vi "TCP Client_34_enablep.vi"(0 "CMD":i32(ring) items=["OCP_IF_CMD_TRACE_READ", "OCP_IF_CMD_TRACE_RESET", "OCP_IF_CMD_TRACE_GET_SIZE", "OCP_IF_CMD_TRACE_SET_SIZE", "OCP_IF_CMD_TRACE_GET_NUMBER_SIGNALS", "OCP_IF_CMD_TRACE_GET_SIGNALS_NAMES", "OCP_IF_CMD_TRACE_GET_NUMBER_TRACES", "OCP_IF_CMD_TRACE_GET_TRACES_NAMES", "OCP_IF_CMD_TRACE_GET_ADDRESS", "OCP_IF_CMD_CS_STATUS", "OCP_IF_CMD_CS_ENABLE", "OCP_IF_CMD_CS_DISABLE", "OCP_IF_CMD_CS_CONTROLLER_IF", "OCP_IF_CMD_CS_HARDWARE_IF", "OCP_IF_CMD_CS_GET_NUMBER_CONTROLLERS", "OCP_IF_CMD_CS_GET_CONTROLLERS_NAMES", "OCP_IF_CMD_PLATFORM_ID", "OCP_IF_CMD_PLATFORM_IF", "OCP_IF_CMD_OPIL_UPDATE_MEASUREMENTS", "OCP_IF_CMD_OPIL_UPDATE_SIM_DATA", "OCP_IF_CMD_OPIL_RUN_CONTROL", "OCP_IF_CMD_OPIL_INITIALIZE_CONTROL", "OCP_IF_CMD_OPIL_GET_CONTROL", "OCP_IF_CMD_OPIL_GET_CONTROLLER_DATA", "OCP_IF_CMD_END"], 1 "CS_IF_Params":T1 {"CS_Duty" min=0 max=1}, 2 "Input Cluster":T4, 3 "error in (no error)":errorcluster, 8 "Comunication Cluster":T2) -> (6 "Output cluster":T3, 7 "R_message 1":string, 10 "error out":errorcluster)   [LabVIEW 2021]
uses:
  <vilib>/ErrorRing/Error Ring.xnode
  <vilib>/Utility/error.llb/Error Cluster From Error Code.vi
panel:
  out "R_Data string length":cluster{i32}
  out "W_Data string length: \nbytes written 2":i32
  out "W_Data string_flat":string
  # "0-> OCP_IF_CMD_TRACE_READ = 0, //LV: SIZE - CMD - ID || RESPONSE: SIZE - DATA\n1->\tOCP_IF_CMD_TRACE_RESET, //SIZE - CMD - ID || RESPONSE: SIZE\n2-> OCP_IF_CMD_TRACE_GET_SIZE, //SIZE - CMD - ID || RESPONSE: SIZE - TRACE_SIZE (4 bztes)\n3->\tOCP_IF_CMD_TRACE_SET_SIZE, //SIZE - CMD - ID - TRACE_SIZE ( 4 bytes) || RESPONSE: SIZE\n4->\tOCP_IF_CMD_TRACE_GET_NUMBER_SIGNALS, //SIZE - CMD - ID || RESPONSE: SIZE - NB_SIGNALS (4 bytes)\n5->\tOCP_IF_CMD_TRACE_GET_SIGNALS_NAMES, //SIZE - CMD - ID || RESPONSE: SIZE - string\n6->\tOCP_IF_CMD_TRACE_GET_NUMBER_TRACES, //SIZE - CMD  || RESPONSE: SIZE - NB_TRACES (4 bytes)\n7->\tOCP_IF_CMD_TRACE_GET_TRACES_NAMES, //SIZE - CMD || RESPONSE: SIZE - NB_TRACES (N bytes)\n8-> OCP_IF_CMD_TRACE_GET_ADDRESS, //SIZE - CMD - ID || RESPONSE: SIZE - TRACE ADDRESS (4 bytes)\n9-> OCP_IF_CMD_CS_STATUS, //SIZE - CMD - ID || RESPONSE: SIZE - CS STATUS (4 bytes)\n10-> OCP_IF_CMD_CS_ENABLE, //SIZE - CMD - ID || RESPONSE: SIZE\n11-> OCP_IF_CMD_CS_DISABLE, //SIZE - CMD - ID || RESPONSE: SIZE\n12-> OCP_IF_CMD_CS_CONTROLLER_IF, //SIZE - CMD - ID - DATA (N) || RESPONSE: SIZE - DATA (M)\n13-> OCP_IF_CMD_CS_HARDWARE_IF, //SIZE - CMD - ID - DATA (N) || RESPONSE: SIZE - DATA (M)\n14-> OCP_IF_CMD_CS_GET_NUMBER_CONTROLLERS, //SIZE - CMD || RESPONSE: SIZE - NB CSs\n15-> OCP_IF_CMD_CS_GET_CONTROLLERS_NAMES, //SIZE - CMD || RESPONSE: SIZE - string NAMES CSs"
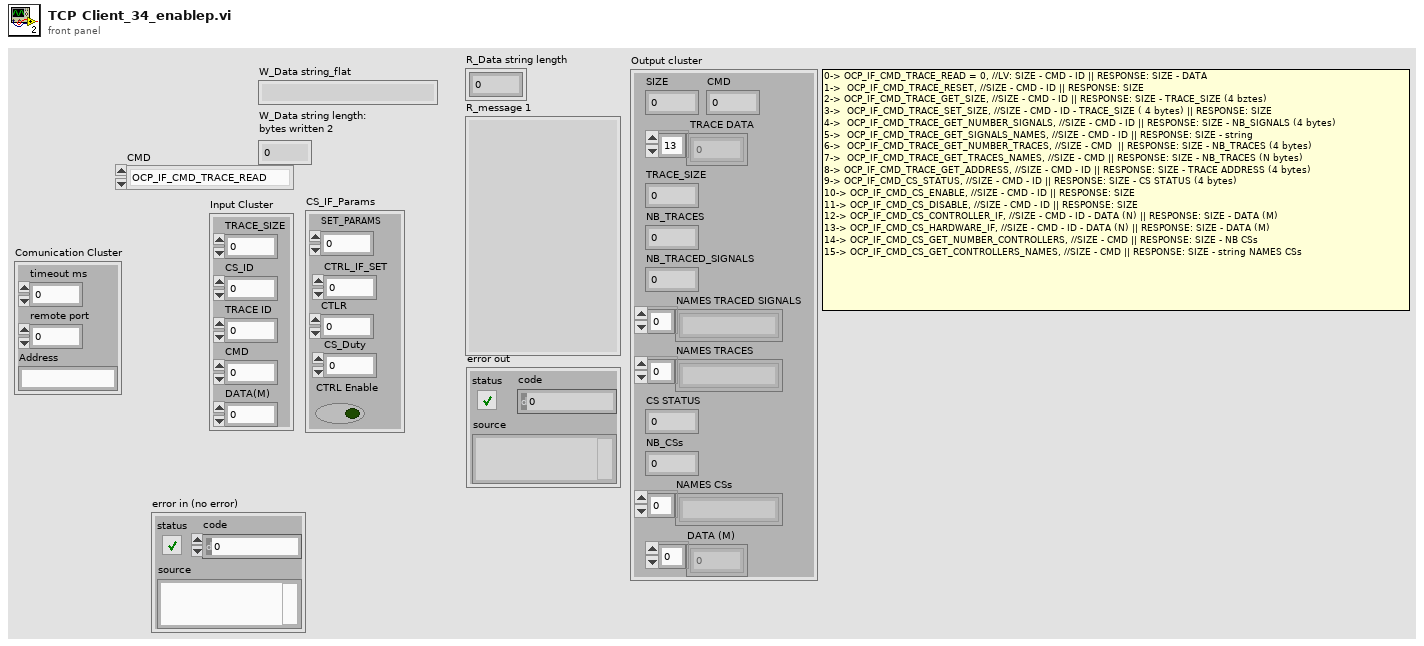
[diagram p1: front panel]
types:
  T1 = cluster{"SET_PARAMS":i32, "CTLR":i32, "CS_Duty":sgl, "CTRL_IF_SET":i32, "CTRL Enable":bool}
  T2 = cluster{"timeout ms":i32, "remote port":u16, "Address":string}
  T3 = cluster{"SIZE":i32, " TRACE DATA":sgl[], "TRACE_SIZE":i32, "NB_TRACES":i32, "NB_TRACED_SIGNALS":i32, "NAMES TRACED SIGNALS":string[], "NAMES TRACES":string[], "CS STATUS":i32, "NB_CSs":i32, "NAMES CSs":string[], "DATA (M)":sgl[], "CMD":i32}
  T4 = cluster{"TRACE_SIZE":i32, "CS_ID":i32, "TRACE ID":i32, "CMD":i32, "DATA(M)":i32}
  T5 = enum16{"big-endian, network order", "native, host order", "little-endian"}
  T6 = enum16{"Standard", "Buffered", "CRLF", "Immediate"}
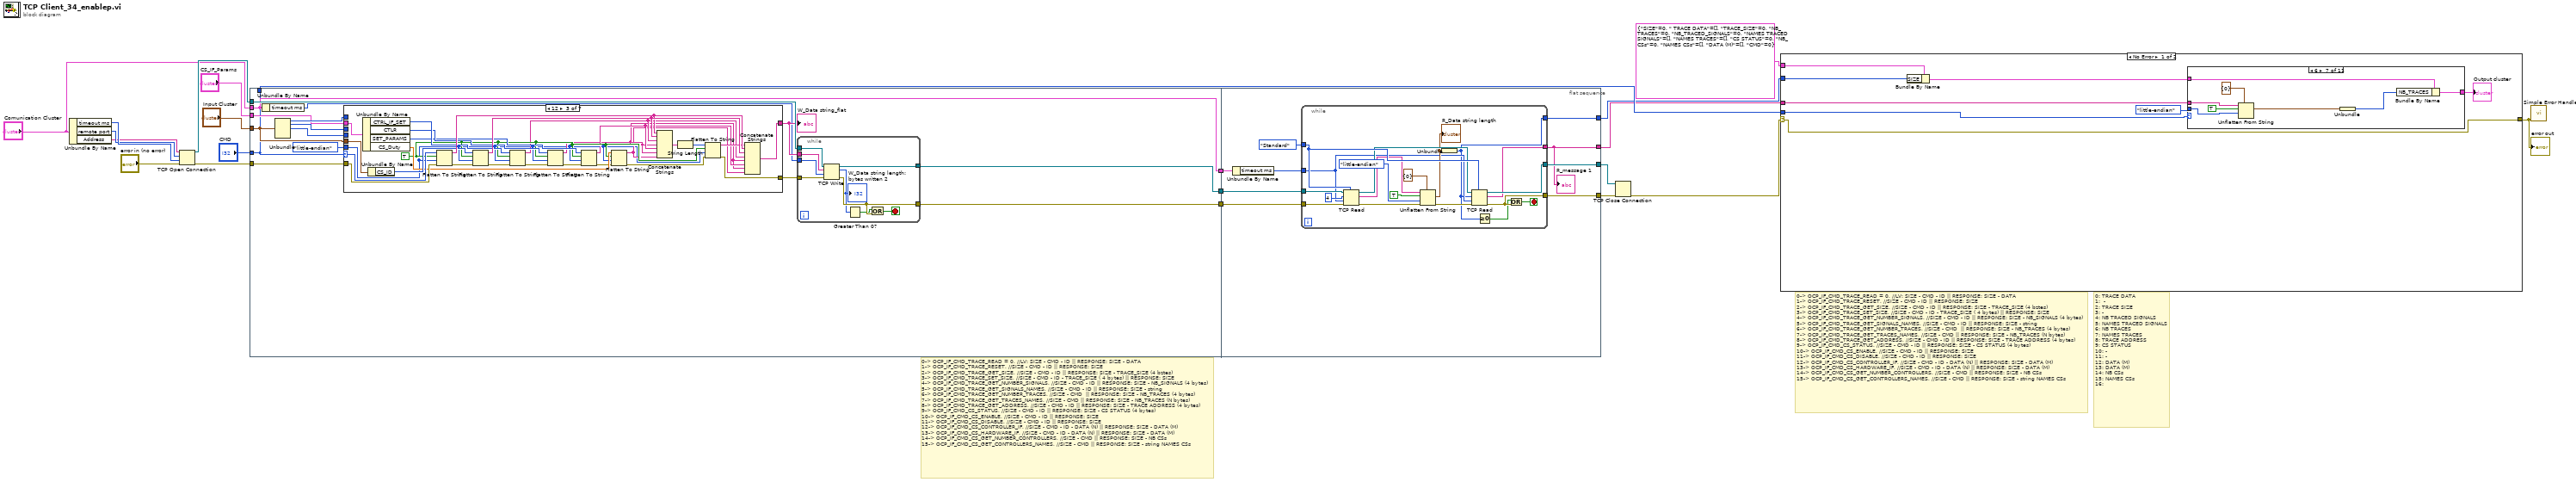
[diagram p0: block diagram]
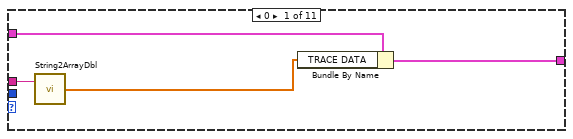
[diagram p2: hidden frame]
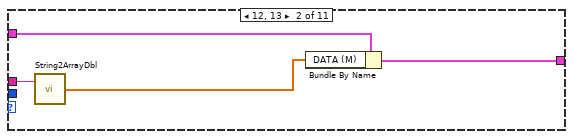
[diagram p3: hidden frame]
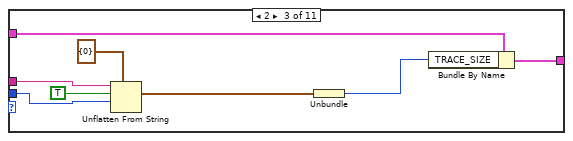
[diagram p4: hidden frame]
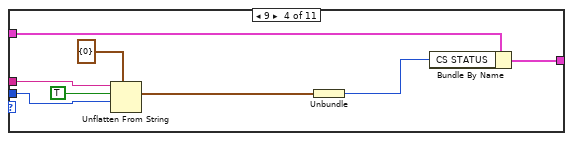
[diagram p5: hidden frame]
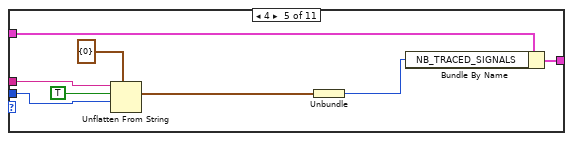
[diagram p6: hidden frame]
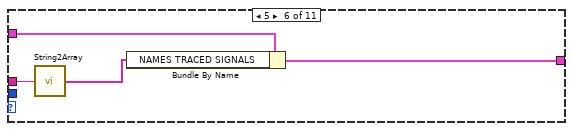
[diagram p7: hidden frame]
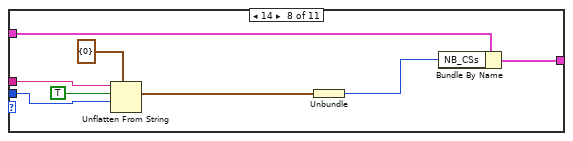
[diagram p8: hidden frame]
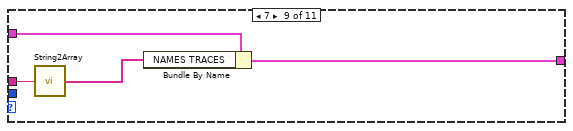
[diagram p9: hidden frame]
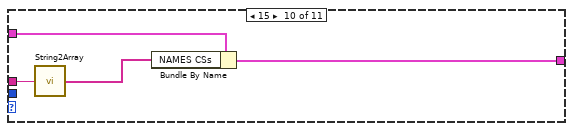
[diagram p10: hidden frame]
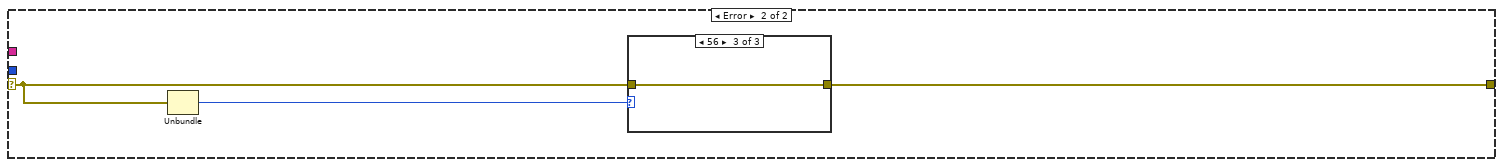
[diagram p12: hidden frame]
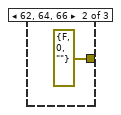
[diagram p14: hidden frame]
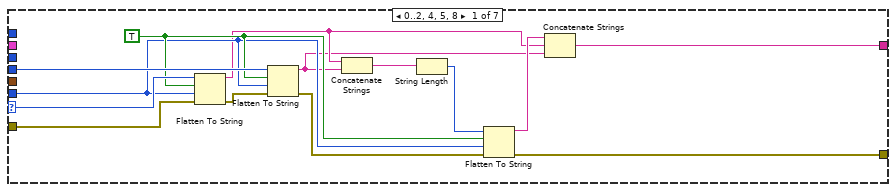
[diagram p15: hidden frame]
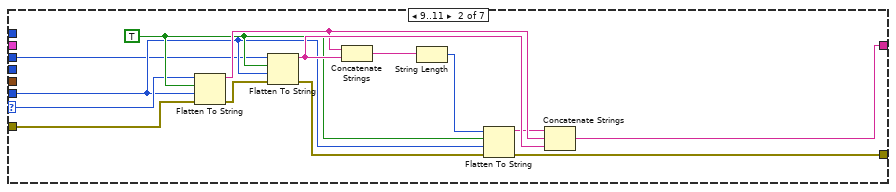
[diagram p16: hidden frame]
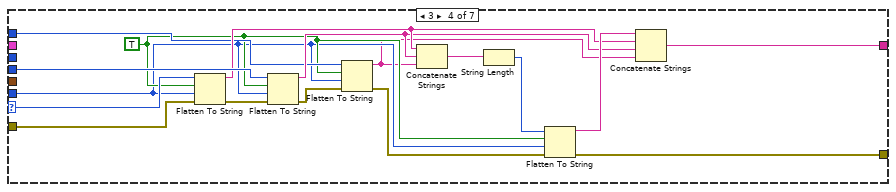
[diagram p17: hidden frame]
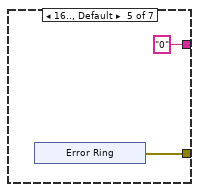
[diagram p18: hidden frame]
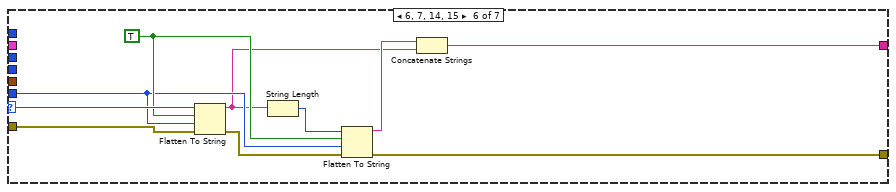
[diagram p19: hidden frame]
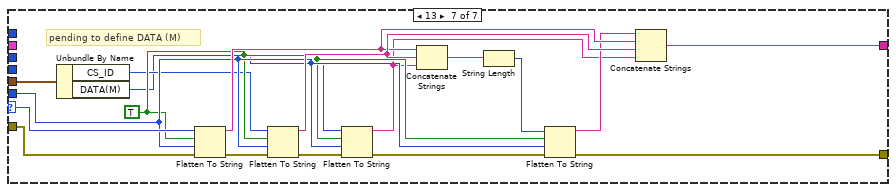
[diagram p20: hidden frame]
diagram:
  # "0-> OCP_IF_CMD_TRACE_READ = 0, //LV: SIZE - CMD - ID || RESPONSE: SIZE - DATA\n1->\tOCP_IF_CMD_TRACE_RESET, //SIZE - CMD - ID || RESPONSE: SIZE\n2-> OCP_IF_CMD_TRACE_GET_SIZE, //SIZE - CMD - ID || RESPONSE: SIZE - TRACE_SIZE (4 bztes)\n3->\tOCP_IF_CMD_TRACE_SET_SIZE, //SIZE - CMD - ID - TRACE_SIZE ( 4 bytes) || RESPONSE: SIZE\n4->\tOCP_IF_CMD_TRACE_GET_NUMBER_SIGNALS, //SIZE - CMD - ID || RESPONSE: SIZE - NB_SIGNALS (4 bytes)\n5->\tOCP_IF_CMD_TRACE_GET_SIGNALS_NAMES, //SIZE - CMD - ID || RESPONSE: SIZE - string\n6->\tOCP_IF_CMD_TRACE_GET_NUMBER_TRACES, //SIZE - CMD  || RESPONSE: SIZE - NB_TRACES (4 bytes)\n7->\tOCP_IF_CMD_TRACE_GET_TRACES_NAMES, //SIZE - CMD || RESPONSE: SIZE - NB_TRACES (N bytes)\n8-> OCP_IF_CMD_TRACE_GET_ADDRESS, //SIZE - CMD - ID || RESPONSE: SIZE - TRACE ADDRESS (4 bytes)\n9-> OCP_IF_CMD_CS_STATUS, //SIZE - CMD - ID || RESPONSE: SIZE - CS STATUS (4 bytes)\n10-> OCP_IF_CMD_CS_ENABLE, //SIZE - CMD - ID || RESPONSE: SIZE\n11-> OCP_IF_CMD_CS_DISABLE, //SIZE - CMD - ID || RESPONSE: SIZE\n12-> OCP_IF_CMD_CS_CONTROLLER_IF, //SIZE - CMD - ID - DATA (N) || RESPONSE: SIZE - DATA (M)\n13-> OCP_IF_CMD_CS_HARDWARE_IF, //SIZE - CMD - ID - DATA (N) || RESPONSE: SIZE - DATA (M)\n14-> OCP_IF_CMD_CS_GET_NUMBER_CONTROLLERS, //SIZE - CMD || RESPONSE: SIZE - NB CSs\n15-> OCP_IF_CMD_CS_GET_CONTROLLERS_NAMES, //SIZE - CMD || RESPONSE: SIZE - string NAMES CSs"
  # "0: TRACE DATA\n1:  -\n2: TRACE SIZE\n3: -\n4: NB TRACED SIGNALS\n5: NAMES TRACED SIGNALS\n6: NB TRACES\n7: NAMES TRACES\n8: TRACE ADDRESS\n9: CS STATUS\n10: -\n11: -\n12: DATA (M)\n13: DATA (M)\n14: NB CSs \n15: NAMES CSs \n16:"
  # "0-> OCP_IF_CMD_TRACE_READ = 0, //LV: SIZE - CMD - ID || RESPONSE: SIZE - DATA\n1->\tOCP_IF_CMD_TRACE_RESET, //SIZE - CMD - ID || RESPONSE: SIZE\n2-> OCP_IF_CMD_TRACE_GET_SIZE, //SIZE - CMD - ID || RESPONSE: SIZE - TRACE_SIZE (4 bztes)\n3->\tOCP_IF_CMD_TRACE_SET_SIZE, //SIZE - CMD - ID - TRACE_SIZE ( 4 bytes) || RESPONSE: SIZE\n4->\tOCP_IF_CMD_TRACE_GET_NUMBER_SIGNALS, //SIZE - CMD - ID || RESPONSE: SIZE - NB_SIGNALS (4 bytes)\n5->\tOCP_IF_CMD_TRACE_GET_SIGNALS_NAMES, //SIZE - CMD - ID || RESPONSE: SIZE - string\n6->\tOCP_IF_CMD_TRACE_GET_NUMBER_TRACES, //SIZE - CMD  || RESPONSE: SIZE - NB_TRACES (4 bytes)\n7->\tOCP_IF_CMD_TRACE_GET_TRACES_NAMES, //SIZE - CMD || RESPONSE: SIZE - NB_TRACES (N bytes)\n8-> OCP_IF_CMD_TRACE_GET_ADDRESS, //SIZE - CMD - ID || RESPONSE: SIZE - TRACE ADDRESS (4 bytes)\n9-> OCP_IF_CMD_CS_STATUS, //SIZE - CMD - ID || RESPONSE: SIZE - CS STATUS (4 bytes)\n10-> OCP_IF_CMD_CS_ENABLE, //SIZE - CMD - ID || RESPONSE: SIZE\n11-> OCP_IF_CMD_CS_DISABLE, //SIZE - CMD - ID || RESPONSE: SIZE\n12-> OCP_IF_CMD_CS_CONTROLLER_IF, //SIZE - CMD - ID - DATA (N) || RESPONSE: SIZE - DATA (M)\n13-> OCP_IF_CMD_CS_HARDWARE_IF, //SIZE - CMD - ID - DATA (N) || RESPONSE: SIZE - DATA (M)\n14-> OCP_IF_CMD_CS_GET_NUMBER_CONTROLLERS, //SIZE - CMD || RESPONSE: SIZE - NB CSs\n15-> OCP_IF_CMD_CS_GET_CONTROLLERS_NAMES, //SIZE - CMD || RESPONSE: SIZE - string NAMES CSs"
  n1 = Unbundle By Name("Comunication Cluster") -> ("timeout ms"=w6:i32, "remote port"=w5:u16, "Address"=w4:string)
  n2 = TCP Open Connection(address=w4, remote port or service name=w5, timeout ms (60000)=w6, error in (no error)="error in (no error)") -> (connection ID=w21:refnum<k5>, error out=w20:errorcluster)  [unwired: 1 in]
  n3 = flat-sequence {
    tunnel: w21 -> [w36]
    tunnel: w20 -> [w33]
    tunnel: [w35] -> w19
    tunnel: [w34] -> w18
    tunnel: [w22] -> w12
    tunnel: "Input Cluster" -> [w27]
    tunnel: "Comunication Cluster" -> [w25]
    tunnel: [w25] -> w3
    tunnel: "CS_IF_Params" -> [w24]
    tunnel: "CMD" -> [w22]
    tunnel: w19 -> [w161]
    tunnel: w18 -> [w160]
    tunnel: [w159] -> w15
    tunnel: [w158] -> w14
    tunnel: [w157] -> w11
    tunnel: [w156] -> w9
    tunnel: w3 -> [w155]
    frame #0 {
      n4 = Unbundle By Name(w25) -> ("timeout ms"=w26:i32)
      n5 = Unbundle(w27) -> ("TRACE_SIZE"=w28:i32, "CS_ID"=w30:i32, "TRACE ID"=w29:i32)  [unwired: 2 out]
      n6 = case shown="12" w22 {
        selector: w22 -> [w57 w64 w94 w116 _ w134 w145]
        tunnel: w33 -> [w59 w65 w95 w118 _ w135 w144]
        tunnel: T5."little-endian" ("byte order (0:big-endian, network order)") -> [w50 w63 w74 w104 _ w130 w141]
        tunnel: w29 -> [w56 _ _ w115 _ _ _]
        tunnel: [w49 w61 w93 w111 "0" w129 w147] -> w32
        tunnel: [w48 w60 w92 w103 w120 w127 w146] -> w31
        tunnel: w28 -> [_ _ _ w106 _ _ _]
        tunnel: w30 -> [_ w62 _ _ _ _ _]
        tunnel: w27 -> [_ _ w91 _ _ _ w143]
        tunnel: w24 -> [_ _ w89 _ _ _ _]
        frame 0..2, 4, 5, 8 {
          w51 = TRUE ("prepend array or string size? (T)")
          n7 = Flatten To String(anything=w57, prepend array or string size? (T)=w51, byte order (0:big-endian, network order)=w50, error in (no error)=w59) -> (data string=w47:string, error out=w58:errorcluster)  [unwired: 1 out]
          n8 = Flatten To String(anything=w56, prepend array or string size? (T)=w51, byte order (0:big-endian, network order)=w50, error in (no error)=w58) -> (data string=w46:string, error out=w53:errorcluster)  [unwired: 1 out]
          n9 = Concatenate Strings(w47, w46) -> (w55:string)
          n10 = String Length(string=w55) -> (length=w54:i32)
          n11 = Flatten To String(anything=w54, prepend array or string size? (T)=w51, byte order (0:big-endian, network order)=w50, error in (no error)=w53) -> (data string=w52:string, error out=w48:errorcluster)  [unwired: 1 out]
          n12 = Concatenate Strings(w52, w47, w46) -> (w49:string)
        }
        frame 9..11 {
          w66 = TRUE ("prepend array or string size? (T)")
          n13 = Flatten To String(anything=w64, prepend array or string size? (T)=w66, byte order (0:big-endian, network order)=w63, error in (no error)=w65) -> (data string=w72:string, error out=w67:errorcluster)  [unwired: 1 out]
          n14 = Flatten To String(anything=w62, prepend array or string size? (T)=w66, byte order (0:big-endian, network order)=w63, error in (no error)=w67) -> (data string=w73:string, error out=w70:errorcluster)  [unwired: 1 out]
          n15 = Concatenate Strings(w72, w73) -> (w68:string)
          n16 = String Length(string=w68) -> (length=w69:i32)
          n17 = Flatten To String(anything=w69, prepend array or string size? (T)=w66, byte order (0:big-endian, network order)=w63, error in (no error)=w70) -> (data string=w71:string, error out=w60:errorcluster)  [unwired: 1 out]
          n18 = Concatenate Strings(w71, w72, w73) -> (w61:string)
        }
        frame 12 {
          w79 = TRUE ("prepend array or string size? (T)")
          n19 = Unbundle By Name(w89) -> ("CTRL_IF_SET"=w87:i32, "CTLR"=w86:i32, "SET_PARAMS"=w84:i32, "CS_Duty"=w83:sgl)
          n20 = Unbundle By Name(w91) -> ("CS_ID"=w90:i32)
          n21 = Flatten To String(anything=w94, prepend array or string size? (T)=w79, byte order (0:big-endian, network order)=w74, error in (no error)=w95) -> (data string=w100:string, error out=w96:errorcluster)  [unwired: 1 out]
          n22 = Flatten To String(anything=w90, prepend array or string size? (T)=w79, byte order (0:big-endian, network order)=w74, error in (no error)=w96) -> (data string=w101:string, error out=w88:errorcluster)  [unwired: 1 out]
          n23 = Flatten To String(anything=w87, prepend array or string size? (T)=w79, byte order (0:big-endian, network order)=w74, error in (no error)=w88) -> (data string=w78:string, error out=w85:errorcluster)  [unwired: 1 out]
          n24 = Flatten To String(anything=w86, prepend array or string size? (T)=w79, byte order (0:big-endian, network order)=w74, error in (no error)=w85) -> (data string=w76:string, error out=w82:errorcluster)  [unwired: 1 out]
          n25 = Flatten To String(anything=w84, prepend array or string size? (T)=w79, byte order (0:big-endian, network order)=w74, error in (no error)=w82) -> (data string=w77:string, error out=w81:errorcluster)  [unwired: 1 out]
          n26 = Flatten To String(anything=w83, prepend array or string size? (T)=w79, byte order (0:big-endian, network order)=w74, error in (no error)=w81) -> (data string=w75:string, error out=w80:errorcluster)  [unwired: 1 out]
          n27 = Concatenate Strings(w100, w101, w78, w76, w77, w76, w75) -> (w97:string)
          n28 = String Length(string=w97) -> (length=w98:i32)
          n29 = Flatten To String(anything=w98, prepend array or string size? (T)=w79, byte order (0:big-endian, network order)=w74, error in (no error)=w80) -> (data string=w99:string, error out=w92:errorcluster)  [unwired: 1 out]
          n30 = Concatenate Strings(w99, w100, w101, w78, w76, w77, w76, w75) -> (w93:string)
        }
        frame 3 {
          w105 = TRUE ("prepend array or string size? (T)")
          n31 = Flatten To String(anything=w116, prepend array or string size? (T)=w105, byte order (0:big-endian, network order)=w104, error in (no error)=w118) -> (data string=w110:string, error out=w117:errorcluster)  [unwired: 1 out]
          n32 = Flatten To String(anything=w115, prepend array or string size? (T)=w105, byte order (0:big-endian, network order)=w104, error in (no error)=w117) -> (data string=w109:string, error out=w108:errorcluster)  [unwired: 1 out]
          n33 = Flatten To String(anything=w106, prepend array or string size? (T)=w105, byte order (0:big-endian, network order)=w104, error in (no error)=w108) -> (data string=w102:string, error out=w107:errorcluster)  [unwired: 1 out]
          n34 = Concatenate Strings(w110, w109, w102) -> (w114:string)
          n35 = String Length(string=w114) -> (length=w113:i32)
          n36 = Flatten To String(anything=w113, prepend array or string size? (T)=w105, byte order (0:big-endian, network order)=w104, error in (no error)=w107) -> (data string=w112:string, error out=w103:errorcluster)  [unwired: 1 out]
          n37 = Concatenate Strings(w112, w110, w109, w102) -> (w111:string)
        }
        frame 16.., Default {
          n38 = xnode "Error Ring"() -> ("error out"=w120:errorcluster)
        }
        frame 6, 7, 14, 15 {
          w131 = TRUE ("prepend array or string size? (T)")
          n39 = Flatten To String(anything=w134, prepend array or string size? (T)=w131, byte order (0:big-endian, network order)=w130, error in (no error)=w135) -> (data string=w126:string, error out=w128:errorcluster)  [unwired: 1 out]
          n40 = String Length(string=w126) -> (length=w133:i32)
          n41 = Flatten To String(anything=w133, prepend array or string size? (T)=w131, byte order (0:big-endian, network order)=w130, error in (no error)=w128) -> (data string=w132:string, error out=w127:errorcluster)  [unwired: 1 out]
          n42 = Concatenate Strings(w132, w126) -> (w129:string)
        }
        frame 13 {
          w140 = TRUE ("prepend array or string size? (T)")
          # "pending to define DATA (M)"
          n43 = Unbundle By Name(w143) -> ("CS_ID"=w139:i32, "DATA(M)"=w138:i32)
          n44 = Flatten To String(anything=w145, prepend array or string size? (T)=w140, byte order (0:big-endian, network order)=w141, error in (no error)=w144) -> (data string=w152:string, error out=w148:errorcluster)  [unwired: 1 out]
          n45 = Flatten To String(anything=w139, prepend array or string size? (T)=w140, byte order (0:big-endian, network order)=w141, error in (no error)=w148) -> (data string=w153:string, error out=w142:errorcluster)  [unwired: 1 out]
          n46 = Flatten To String(anything=w138, prepend array or string size? (T)=w140, byte order (0:big-endian, network order)=w141, error in (no error)=w142) -> (data string=w137:string, error out=w136:errorcluster)  [unwired: 1 out]
          n47 = Concatenate Strings(w152, w153, w137) -> (w149:string)
          n48 = String Length(string=w149) -> (length=w150:i32)
          n49 = Flatten To String(anything=w150, prepend array or string size? (T)=w140, byte order (0:big-endian, network order)=w141, error in (no error)=w136) -> (data string=w151:string, error out=w146:errorcluster)  [unwired: 1 out]
          n50 = Concatenate Strings(w151, w152, w153, w137) -> (w147:string)
        }
      }
      "W_Data string_flat" <- w32
      n51 = while {
        tunnel: w32 -> [w43]
        tunnel: w26 -> [w41]
        tunnel: w36 -> [w45]
        tunnel: [w44] -> w34
        tunnel: w31 -> [w42]
        tunnel: [w39] -> w35
        stop <- w40 stop-if-true
        n52 = TCP Write(connection ID=w45, data in=w43, error in (no error)=w42, 9:w41) -> (connection ID out=w44:refnum<k5>, bytes written=w37:i32, error out=w39:errorcluster)
        "W_Data string length: \nbytes written 2" <- w37
        n53 = Greater Than 0?(x=w37) -> (x > 0?=w38:bool)
        n54 = Or(x=w38, y=w39) -> (x .or. y?=w40:bool)
      }
    }
    frame #1 {
      n55 = Unbundle By Name(w155) -> ("timeout ms"=w154:i32)
      n56 = while {
        tunnel: T6."Standard" ("mode (standard)") -> [w181]
        tunnel: [w169] -> w157
        tunnel: [w164] -> w156
        tunnel: w154 -> [w168]
        tunnel: w160 -> [w178]
        tunnel: [w177] -> w159
        tunnel: w161 -> [w179]
        tunnel: [w165] -> w158
        stop <- w166 stop-if-true
        n57 = TCP Read(connection ID=w178, bytes to read=4, error in (no error)=w179, 7:w181, 9:w168) -> (connection ID out=w180:refnum<k5>, data out=w176:string, error out=w172:errorcluster)
        n58 = Unflatten From String(type=cluster{i32} {0}, binary string=w176, data includes array or string size? (T)=TRUE, byte order (0:big-endian, network order)=T5."little-endian", error in (no error)=w172) -> (value=w173:cluster{i32}, error out=w171:errorcluster)  [unwired: 1 out]
        "R_Data string length" <- w173
        n59 = Unbundle(w173) -> (w164:i32)
        n60 = TCP Read(connection ID=w180, bytes to read=w164, error in (no error)=w171, 7:w181, 9:w168) -> (connection ID out=w177:refnum<k5>, data out=w169:string, error out=w165:errorcluster)
        n61 = Greater Or Equal To 0?(x=w164) -> (x >= 0?=w163:bool)
        n62 = Or(x=w163, y=w165) -> (x .or. y?=w166:bool)
      }
      "R_message 1" <- w157
    }
  }
  n63 = TCP Close Connection(connection ID=w15, error in (no error)=w14) -> (error out=w16:errorcluster)  [unwired: 1 in, 1 out]
  n64 = case shown="No Error" w16 {
    selector: w16 -> [w189 w252]
    tunnel: [w189 w251] -> w17
    tunnel: w12 -> [w184 _]
    tunnel: w11 -> [w185 _]
    tunnel: T3 {"SIZE"=0, " TRACE DATA"=[], "TRACE_SIZE"=0, "NB_TRACES"=0, "NB_TRACED_SIGNALS"=0, "NAMES TRACED SIGNALS"=[], "NAMES TRACES"=[], "CS STATUS"=0, "NB_CSs"=0, "NAMES CSs"=[], "DATA (M)"=[], "CMD"=0} ("input cluster") -> [w188 _]
    tunnel: w9 -> [w186 _]
    frame No Error {
      n65 = Bundle By Name(cluster=w188, "SIZE"=w186) -> (w187:T3)
      n66 = case shown="6" w184 {
        tunnel: [w192 w196 w204 w212 w220 w224 w233 w241 w244 w248 w250] -> w183
        tunnel: w187 -> [w193 w197 w205 w213 w221 w225 w230 w238 w245 w249 w250]
        tunnel: w185 -> [w190 w194 w202 w210 w217 w223 w228 w236 w243 w247 _]
        tunnel: T5."little-endian" ("byte order (0:big-endian, network order)") -> [_ _ w200 w208 w216 _ w229 w237 _ _ _]
        frame 0 {
          n67 = call "String2ArrayDbl.vi"("R_message 1"=w190) -> ("Array"=w191:sgl[])  [unwired: 1 in]
          n68 = Bundle By Name(cluster=w193, "TRACE DATA"=w191) -> (w192:T3)
        }
        frame 12, 13 {
          n69 = call "String2ArrayDbl.vi"("R_message 1"=w194) -> ("Array"=w195:sgl[])  [unwired: 1 in]
          n70 = Bundle By Name(cluster=w197, "DATA (M)"=w195) -> (w196:T3)
        }
        frame 2 {
          n71 = Unflatten From String(type=cluster{i32} {0}, binary string=w202, data includes array or string size? (T)=TRUE, byte order (0:big-endian, network order)=w200) -> (value=w199:cluster{i32})  [unwired: 1 in, 2 out]
          n72 = Unbundle(w199) -> (w198:i32)
          n73 = Bundle By Name(cluster=w205, "TRACE_SIZE"=w198) -> (w204:T3)
        }
        frame 9 {
          n74 = Unflatten From String(type=cluster{i32} {0}, binary string=w210, data includes array or string size? (T)=TRUE, byte order (0:big-endian, network order)=w208) -> (value=w207:cluster{i32})  [unwired: 1 in, 2 out]
          n75 = Unbundle(w207) -> (w206:i32)
          n76 = Bundle By Name(cluster=w213, "CS STATUS"=w206) -> (w212:T3)
        }
        frame 4 {
          n77 = Unflatten From String(type=cluster{i32} {0}, binary string=w217, data includes array or string size? (T)=TRUE, byte order (0:big-endian, network order)=w216) -> (value=w218:cluster{i32})  [unwired: 1 in, 2 out]
          n78 = Unbundle(w218) -> (w214:i32)
          n79 = Bundle By Name(cluster=w221, "NB_TRACED_SIGNALS"=w214) -> (w220:T3)
        }
        frame 5 {
          n80 = call "String2Array.vi"("R_message 1"=w223) -> ("Array 2"=w222:string[])
          n81 = Bundle By Name(cluster=w225, "NAMES TRACED SIGNALS"=w222) -> (w224:T3)
        }
        frame 6 {
          n82 = Unflatten From String(type=cluster{i32} {0}, binary string=w228, data includes array or string size? (T)=TRUE, byte order (0:big-endian, network order)=w229) -> (value=w232:cluster{i32})  [unwired: 1 in, 2 out]
          n83 = Unbundle(w232) -> (w226:i32)
          n84 = Bundle By Name(cluster=w230, "NB_TRACES"=w226) -> (w233:T3)
        }
        frame 14 {
          n85 = Unflatten From String(type=cluster{i32} {0}, binary string=w236, data includes array or string size? (T)=TRUE, byte order (0:big-endian, network order)=w237) -> (value=w240:cluster{i32})  [unwired: 1 in, 2 out]
          n86 = Unbundle(w240) -> (w234:i32)
          n87 = Bundle By Name(cluster=w238, "NB_CSs"=w234) -> (w241:T3)
        }
        frame 7 {
          n88 = call "String2Array.vi"("R_message 1"=w243) -> ("Array 2"=w242:string[])
          n89 = Bundle By Name(cluster=w245, "NAMES TRACES"=w242) -> (w244:T3)
        }
        frame 15 {
          n90 = call "String2Array.vi"("R_message 1"=w247) -> ("Array 2"=w246:string[])
          n91 = Bundle By Name(cluster=w249, "NAMES CSs"=w246) -> (w248:T3)
        }
        frame 8, Default {
        }
      }
      "Output cluster" <- w183
    }
    frame Error {
      n92 = Unbundle(w252) -> ("code"=w253:i32)  [unwired: 2 out]
      n93 = case shown="56" w253 {
        tunnel: [w254 errorcluster {"status"=FALSE, "code"=0, "source"=""} ("error IO") w256] -> w251
        tunnel: w252 -> [w254 _ w256]
        frame 0, Default {
        }
        frame 62, 64, 66 {
        }
        frame 56 {
        }
      }
    }
  }
  "error out" <- w17
  n94 = call <vilib>:"Simple Error Handler.vi"("error in (no error)"=w17) -> ()  [unwired: 4 in, 5 out]
